vi "Modules - Create Test.vi"(8 "error in":errorcluster, 11 "Station":string[](array[string])) -> (0 "error out":errorcluster, 2 "Cancel out":bool, 3 "Stations":string)   [LabVIEW 2019]
uses:
  Controls/Create test-state.ctl
  Controls/eFGV States.ctl
  Controls/FGV States.ctl
panel:
  in  "Select Available Test Station :":u16(ring) items=["Please Select...", "TEST"]
  in  "OK":bool
  in  "Cancel":bool
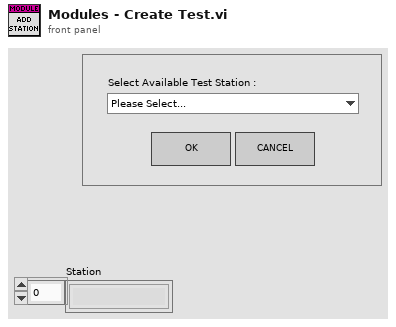
[diagram p1: front panel]
types:
  T1 = typedef "Create test-state.ctl" = enum16{"Init", "Idle", "Select", "Load", "Close", "Exit"}
  T2 = typedef "eFGV States.ctl" = enum16{"Init", "Read", "Write", "Exit"}
  T3 = typedef "FGV States.ctl" = enum16{"Read", "Write"}
  T4 = cluster{"Station Name":string, "Key Value":string[], "Key Names":string[]}[]
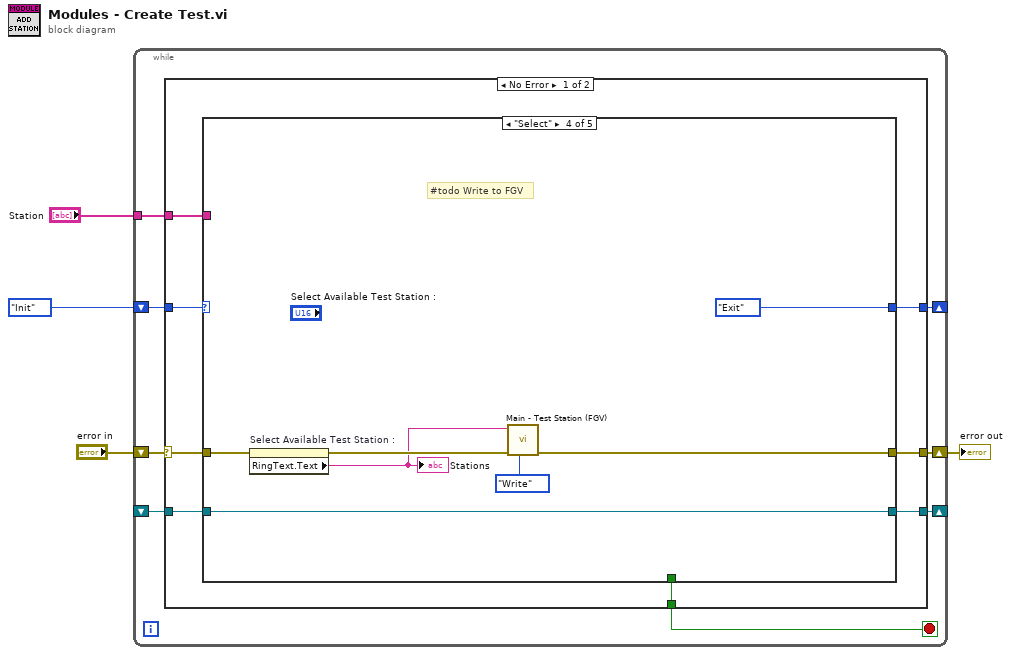
[diagram p0: block diagram]
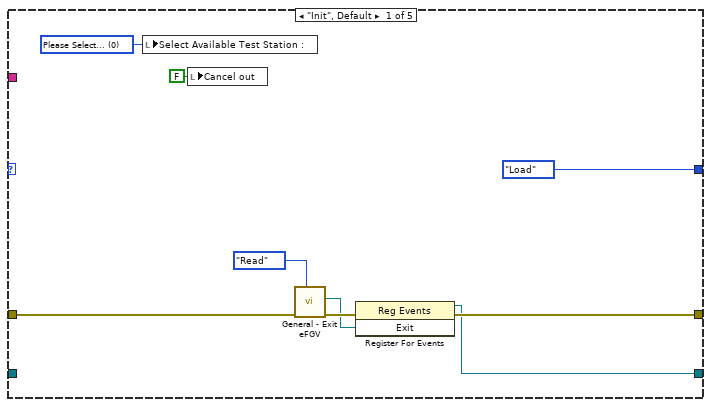
[diagram p2: hidden frame]
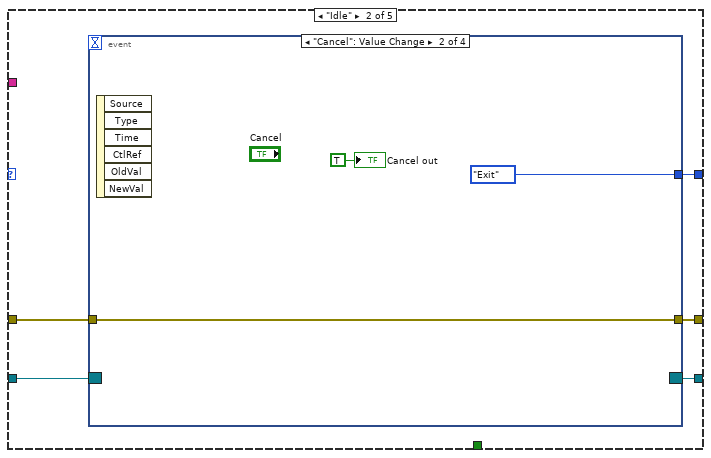
[diagram p3: hidden frame]
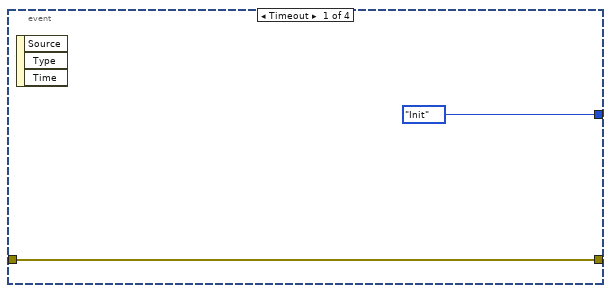
[diagram p4: hidden frame]
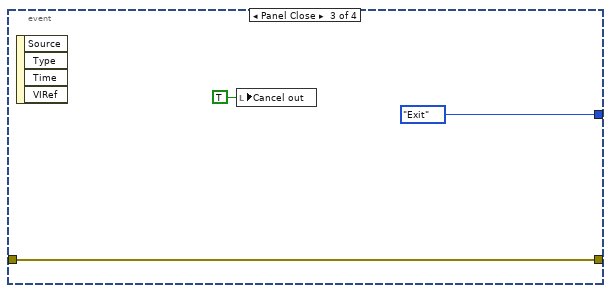
[diagram p5: hidden frame]
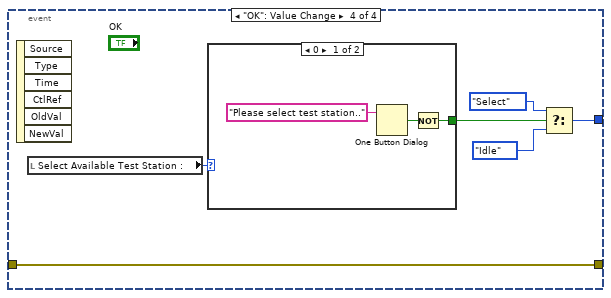
[diagram p6: hidden frame]
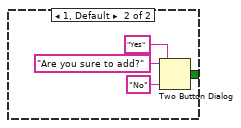
[diagram p7: hidden frame]
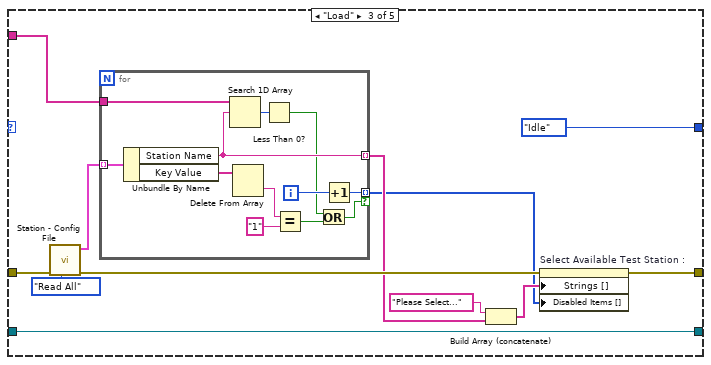
[diagram p8: hidden frame]
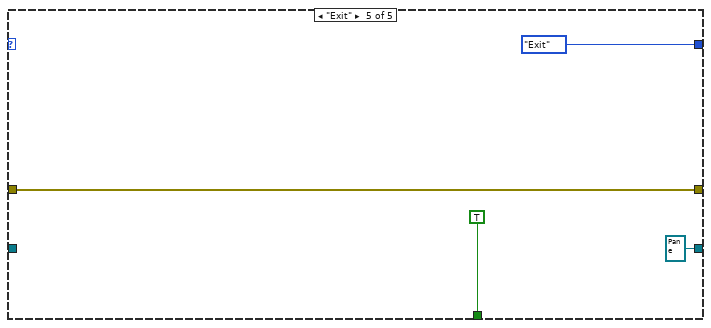
[diagram p9: hidden frame]
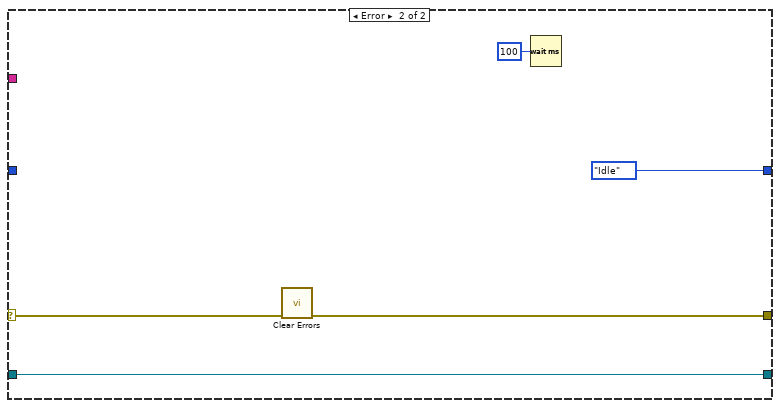
[diagram p10: hidden frame]
diagram:
  n1 = while {
    shift-right: [w11] -> w2
    shift-left: "error in" -> [w12]
    shift-right: [w9] -> _
    shift-left: Create_test-state."Init" -> [w10]
    shift-right: [w7] -> _
    shift-left: _ -> [w6]
    tunnel: "Station" -> [w5]
    stop <- w8 stop-if-true
    n2 = case shown="No Error" w12 {
      selector: w12 -> [w19 w95]
      tunnel: [w18 w93] -> w11
      tunnel: w10 -> [w20 _]
      tunnel: [w17 Create_test-state."Idle"] -> w9
      tunnel: [w16 _] -> w8
      tunnel: [w15 w91] -> w7
      tunnel: w6 -> [w14 w91]
      tunnel: w5 -> [w13 _]
      frame No Error {
        n3 = case shown="\"Select\"" w20 {
          tunnel: w19 -> [w23 w32 w62 w85 w88]
          tunnel: [w24 w34 w66 w80 w88] -> w18
          tunnel: [Create_test-state."Load" w33 Create_test-state."Idle" Create_test-state."Exit" Create_test-state."Exit"] -> w17
          tunnel: [_ _ _ _ TRUE] -> w16
          tunnel: [w21 w30 w57 w81 refnum<event-registration> refnum ("Event Registration Refnum")] -> w15
          tunnel: w14 -> [_ w31 w57 w81 _]
          tunnel: w13 -> [_ _ w56 _ _]
          frame "Init", Default {
            w28 = u16 0 items=["Please Select..."] ("Select Available Test Station :")
            n4 = local write "Select Available Test Station :"(w28) -> ()
            n5 = local write "Cancel out"(FALSE ("Cancel 2")) -> ()
            n6 = call "General - Exit eFGV.vi"("eFGV States"=eFGV_States."Read", "error in (no error)"=w23) -> ("error out"=w26:errorcluster, "Exit"=w25:refnum<user-event>)  [unwired: 7 in, 1 out]
            n7 = register-events(error in=w26, w25) -> (reference out=w21:refnum<event-registration>, error out=w24:errorcluster)  [unwired: 1 in]
          }
          frame "Idle" {
            n8 = event shown="[1] \"Cancel\": Value Change" {
              selector: w31 -> [_ _ _ _]
              dyn-events: [_ _ _ _] -> w30
              timeout: _ -> [_ _ _ _]
              tunnel: w32 -> [w36 w39 w42 w48]
              tunnel: [w36 w39 w42 w48] -> w34
              tunnel: [Create_test-state."Init" Create_test-state."Exit" Create_test-state."Exit" w45] -> w33
              event Timeout {
                n9 = event-data() -> ()  [unwired: 1 in, 3 out]
              }
              event "Cancel": Value Change {
                n10 = event-data() -> ()  [unwired: 1 in, 6 out]
                "Cancel out" <- TRUE ("Cancel 2")
              }
              event Panel Close {
                n11 = event-data() -> ()  [unwired: 1 in, 4 out]
                n12 = local write "Cancel out"(TRUE ("Cancel out")) -> ()
              }
              event "OK": Value Change {
                n13 = event-data() -> ()  [unwired: 1 in, 6 out]
                n14 = local read "Select Available Test Station :"() -> (w43:u16)
                n15 = case shown="0" w43 {
                  tunnel: [w50 w52] -> w44
                  frame 0 {
                    n16 = One Button Dialog(message="Please select test station..") -> (true=w51:bool)  [unwired: 1 in]
                    n17 = Not(x=w51) -> (.not. x?=w50:bool)
                  }
                  frame 1, Default {
                    n18 = Two Button Dialog(message="Are you sure to add?", 1:"No" ("F button name (\"Cancel\")"), 2:"Yes" ("T button name (\"OK\")")) -> (T button?=w52:bool)
                  }
                }
                n19 = Select(t=Create_test-state."Select", s=w44, f=Create_test-state."Idle") -> (s? t:f=w45:T1)
              }
            }
          }
          frame "Load" {
            n20 = call "Station - Config File.vi"("Action"=enum16{"Write", "Read", "Read All", "Remove"}."Read All", "error in (no error)"=w62) -> ("error out"=w61:errorcluster, "Value Out"=w60:T4)  [unwired: 8 in]
            n21 = for {
              tunnel: w60 -> [w79] mode=indexing
              tunnel: [w72] -> w59 mode=indexing
              tunnel: [w76] -> w58 mode=indexing if=w68
              tunnel: w56 -> [w73]
              i -> [w77]
              n22 = Unbundle By Name(w79) -> ("Station Name"=w72:string, "Key Value"=w78:string[])
              n23 = Search 1D Array(1D array=w73, element=w72) -> (index of element=w71:i32)  [unwired: 1 in]
              n24 = Delete From Array(array=w78) -> (deleted portion=w75:string)  [unwired: 2 in, 1 out]
              n25 = Less Than 0?(x=w71) -> (x < 0?=w69:bool)
              n26 = Equal?(x=w75, y="1") -> (x = y?=w70:bool)
              n27 = Or(x=w69, y=w70) -> (x .or. y?=w68:bool)
              n28 = Increment(x=w77) -> (x+1=w76:i32)
            }
            n29 = Build Array (concatenate)("Please Select..." ("String"), w59) -> (w64:string[])
            n30 = property on="Select Available Test Station :" class="Ring (strict)"(error in=w61, "Strings []"=w64, "Disabled Items []"=w58) -> (error out=w66:errorcluster)  [unwired: 1 in, 1 out]
          }
          frame "Select" {
            # "#todo Write to FGV"
            n31 = property on="Select Available Test Station :" class="Ring (strict)"(error in=w85) -> (error out=w84:errorcluster, "RingText.Text"=w82:string)  [unwired: 1 in, 1 out]
            "Stations" <- w82
            n32 = call "Main - Test Station (FGV).vi"("Action"=FGV_States."Write", "error In"=w84, "Station Name"=w82) -> ("error out"=w80:errorcluster)  [unwired: 7 in, 1 out]
          }
          frame "Exit" {
          }
        }
      }
      frame Error {
        n33 = call <vilib>:"Clear Errors.vi"("error in (no error)"=w95) -> ("error out"=w93:errorcluster)  [unwired: 5 in, 1 out]
        n34 = Wait (ms)(milliseconds to wait=u32 100) -> ()  [unwired: 1 out]
      }
    }
  }
  "error out" <- w2
